vi "Write to Lights.vi"   [LabVIEW 2015]
uses:
  Common Code/Shooter State.ctl
  <vilib>/Rock Robotics/WPI/DriverStation/WPI_DriverStationRobotMode2.ctl
  <vilib>/Rock Robotics/WPI/DriverStation/WPI_DriverStationAllianceInfo.ctl
  Common Code/Utilities/TimeManager.vi
  Common Code/Change Detect.vi
  Common Code/Change Detect Boolean.vi
  Robot Global Data.vi
types:
  T1 = typedef "WPI_DriverStationAllianceInfo.ctl" = enum16{"Red", "Blue", "Invalid"}
  T2 = typedef "Shooter State.ctl" = enum16{"Idle", "Settle Ball", "Warmup", "Shooter Ready", "Shoot"}
  T3 = typedef "WPI_DriverStationRobotMode2.ctl" = enum16{"Autonomous Disabled", "Autonomous Enabled", "Teleop Disabled", "Teleop Enabled", "Disconnected", "Finish", "Test Disabled", "Test Enabled", "Emergency Stopped"}
  T4 = typedef "Drivetrain Status Cluster.ctl" = cluster{"Modes":T5, "Y (Throttle)":dbl, "X (Steer)":dbl, "Gyro In Range?":bool, "Distance Drive Finished?":bool, "Stop Eject Lockout":bool, "Dist Drive Status":T6, "Y Target":dbl, "Heading Target":dbl, "Vision Target Aligned?":bool, "Gear":dbl, "1st Gear Time":dbl, "2nd Gear Time":dbl, "1st Gear Shifts":dbl, "2nd Gear Shifts":dbl}
  T5 = typedef "Drivetrain Modes.ctl" = enum16{"Tank", "Climb", "Manual", "Goal Vision Targeting", "PID Distance Drive", "Hybrid", "Gyro Steer"}
  T6 = typedef "Dist Drive Status.ctl" = cluster{"Y In Range":bool, "X In Range":bool, "Gyro In Range":bool, "Y Dist":dbl, "X Dist":dbl, "Gyro":dbl}
  T7 = typedef "Shooter State Cluster.ctl" = cluster{"State":T2, "Left RPM":dbl, "Right RPM":dbl, "Shooter Ready?":bool, "Ball Loaded?":bool, "Current Angle":dbl, "Angle Motor Output":dbl, "Trigger Output":dbl, "Angle Ready?":bool, "RPM Ready?":bool, "Vision Ready?":bool, "Ball Loaded?":bool, "Mode":T8, "Shot Type":T9, "Pot Height":dbl, "Current Tripped Forward?":bool, "Current Tripped Backward?":bool, "Right Servo":i32, "Left Servo":i32, "IR Override":bool, "Intake Danger?":bool, "Intake Angle Ready?":bool}
  T8 = typedef "Shoot Modes Enum.ctl" = enum16{"Manual", "Safe", "Auto"}
  T9 = typedef "Shot Type.ctl" = enum16{"Batter Shot", "Corner Shot", "Cleat Shot", "Vision Shot", "Deep Middle Shot"}
  T10 = typedef "WPI_AOChannelDevRef.ctl" = cluster{"DevStatus":errorcluster, "AO Channel":T11}
  T11 = typedef "WPI_AnalogOutputChannel.ctl" = enum8{"AO MXP 0", "AO MXP 1", "Invalid"}
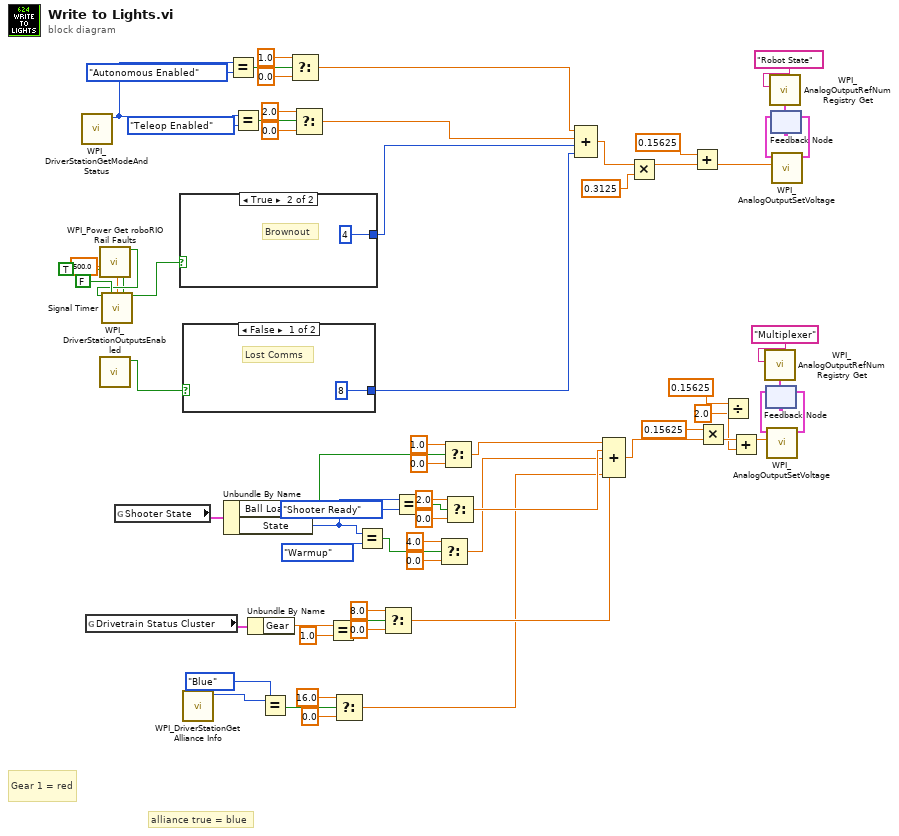
[diagram p0: block diagram]
diagram:
  # "alliance true = blue"
  # "Gear 1 = red"
  n1 = call <vilib>:"WPI_DriverStationGetModeAndStatus.vi"() -> ("Robot Mode"=w28:T3)  [unwired: 10 in, 1 out]
  n2 = global read "Robot Global Data.vi" "Drivetrain Status Cluster"() -> (w46:T4)
  n3 = call <vilib>:"WPI_Power Get roboRIO Rail Faults.vi"() -> ("Input Voltage Brown Out"=w59:bool)  [unwired: 10 in, 5 out]
  n4 = call <vilib>:"WPI_DriverStationOutputsEnabled.vi"() -> ("OutputsEnabled?"=w54:bool)  [unwired: 10 in, 1 out]
  n5 = call "Signal Timer.vi"("Input"=w59, "Edge"=FALSE, "Interval"=500.0, "Pull"=TRUE) -> ("Filtered Output"=w57:bool)  [unwired: 11 in]
  n6 = global read "Robot Global Data.vi" "Shooter State"() -> (w47:T7)
  n7 = case shown="True" w57 {
    tunnel: [_ 4] -> w53
    frame False {
    }
    frame True {
      # "Brownout"
    }
  }
  n8 = case shown="False" w54 {
    tunnel: [8 _] -> w52
    frame False {
      # "Lost Comms"
    }
    frame True {
    }
  }
  n9 = call <vilib>:"WPI_DriverStationGet Alliance Info.vi"() -> ("Alliance"=w6:T1)  [unwired: 10 in, 1 out]
  n10 = Unbundle By Name(w47) -> ("Ball Loaded?"=w43:bool, "State"=w44:T2)
  n11 = Equal?(x=w28, y=WPI_DriverStationRobotMode2."Autonomous Enabled") -> (x = y?=w26:bool)
  n12 = Equal?(x=w28, y=WPI_DriverStationRobotMode2."Teleop Enabled") -> (x = y?=w25:bool)
  n13 = Unbundle By Name(w46) -> ("Gear"=w34:dbl)
  n14 = Equal?(x=w6, y=WPI_DriverStationAllianceInfo."Blue") -> (x = y?=w4:bool)
  n15 = Select(t=1.0, s=w26, f=0.0) -> (s? t:f=w20:dbl)
  n16 = Select(t=2.0, s=w25, f=0.0) -> (s? t:f=w19:dbl)
  n17 = Equal?(x=w34, y=1.0) -> (x = y?=w32:bool)
  n18 = Select(t=16.0, s=w4, f=0.0) -> (s? t:f=w1:dbl)
  n19 = Equal?(x=w44, y=Shooter_State."Warmup") -> (x = y?=w37:bool)
  n20 = Select(t=8.0, s=w32, f=0.0) -> (s? t:f=w15:dbl)
  n21 = Equal?(x=w44, y=Shooter_State."Shooter Ready") -> (x = y?=w40:bool)
  n22 = Select(t=4.0, s=w37, f=0.0) -> (s? t:f=w16:dbl)
  n23 = Select(t=1.0, s=w43, f=0.0) -> (s? t:f=w18:dbl)
  n24 = Select(t=2.0, s=w40, f=0.0) -> (s? t:f=w17:dbl)
  n25 = Compound Arithmetic op=ADD(w20, w19, w53, w52) -> (w55:dbl)
  n26 = Compound Arithmetic op=ADD(w18, w17, w16, w15, w1) -> (w14:dbl)
  n27 = Multiply(x=w55, y=0.3125) -> (x*y=w51:dbl)
  n28 = Add(x=0.15625, y=w51) -> (x+y=w49:dbl)
  n29 = Multiply(x=0.15625, y=w14) -> (x*y=w13:dbl)
  n30 = Divide(x=0.15625 ("y"), y=2.0) -> (x/y=w8:dbl)
  n31 = Add(x=w13, y=w8) -> (x+y=w11:dbl)
  n32 = call <vilib>:"WPI_AnalogOutputRefNum Registry Get.vi"("refnum name"="Multiplexer") -> ("AODeviceRef"=w63:T10)  [unwired: 9 in, 1 out]
  n33 = feedback #1(w63) -> (w62:T10)
  n34 = call <vilib>:"WPI_AnalogOutputSetVoltage.vi"("Voltage"=w11, "AODeviceRef"=w62) -> ("AODeviceRef"=w64:T10)  [unwired: 8 in, 1 out]
  n35 = feedback-in #1(w64) -> ()
  n36 = call <vilib>:"WPI_AnalogOutputRefNum Registry Get.vi"("refnum name"="Robot State") -> ("AODeviceRef"=w67:T10)  [unwired: 9 in, 1 out]
  n37 = feedback #2(w67) -> (w66:T10)
  n38 = call <vilib>:"WPI_AnalogOutputSetVoltage.vi"("Voltage"=w49, "AODeviceRef"=w66) -> ("AODeviceRef"=w68:T10)  [unwired: 8 in, 1 out]
  n39 = feedback-in #2(w68) -> ()
